vi "get_bit.vi"(0 "Position":u16, 1 "INFO":u8[](array[numeric])) -> (2 "Bit_Value":bool, 3 "Byte_index":u16, 4 "Bit_index":u16)   [LabVIEW 2022 SP3]
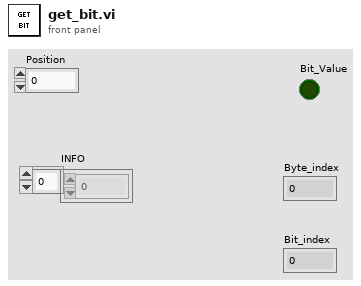
[diagram p1: front panel]
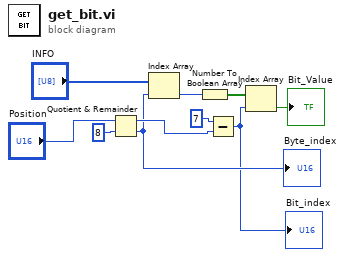
[diagram p0: block diagram]
diagram:
  n1 = Quotient & Remainder(x="Position", y=u16 8) -> (x-y*floor(x/y)=w3:u16, floor(x/y)=w2:u16)
  "Byte_index" <- w2
  n2 = Index Array(array="INFO", index=w2) -> (element=w7:u8)
  n3 = Number To Boolean Array(number=w7) -> (Boolean array=w6:bool[])
  n4 = Subtract(x=u16 7, y=w3) -> (x-y=w1:u16)
  "Bit_index" <- w1
  n5 = Index Array(array=w6, index=w1) -> (element=→"Bit_Value":bool)
